vi "Write Abort Notifier.vi"(8 "error in (no error)":errorcluster, 10 "Abort Notifier":refnum<notifier>, 11 "Slave Test Runner In":refnum<class "Slave Test Runner.lvclass">) -> (0 "error out":errorcluster, 3 "Slave Test Runner Out":refnum<class "Slave Test Runner.lvclass">)   [LabVIEW 2020, in "Slave Test Runner.lvclass"]
uses:
  Slave Test Runner.lvclass
  Slave Test Runner.lvclass/Slave Test Runner.ctl
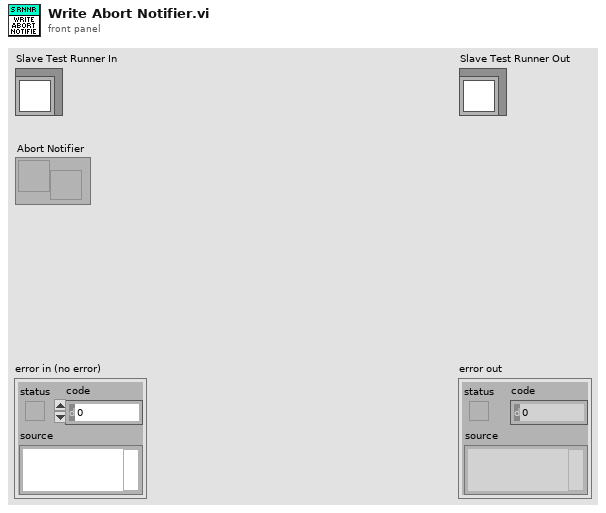
[diagram p1: front panel]
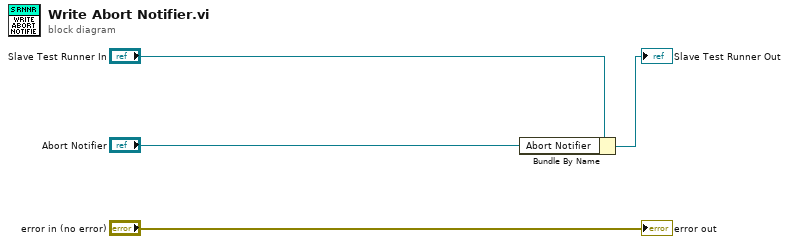
[diagram p0: block diagram]
diagram:
  n1 = Bundle By Name(cluster="Slave Test Runner In", "Abort Notifier"="Abort Notifier") -> (→"Slave Test Runner Out":refnum<class "Slave Test Runner.lvclass">)
  "error out" <- "error in (no error)"
